vi "Initialize.vi"(8 "error in (no error)":errorcluster, 9 "Reset (T: Reset)":bool=TRUE, 10 "ID Query (T: Check)":bool=TRUE, 11 "VISA resource name":refnum<visa-resource-name>) -> (0 "error out":errorcluster, 3 "VISA resource name out":refnum<visa-resource-name>)   [LabVIEW 2015, in "Chroma ATE 6310.lvlib"]
doc: "This VI passes the addressing information in the instrument decriptor to the Instr Open VI and returns the instrument ID. You can optionally reset the instrument by setting the front panel reset control. You must run this VI before using any of the instrument driver VIs for this instrument."
uses:
  <instrlib>/Chroma ATE 6310/Chroma ATE 6310.lvlib
panel:
  # "© 2005 National Instruments.  ALL RIGHTS RESERVED."
  # "Check\nDon't Check"
  # "Reset\nDon't Reset"
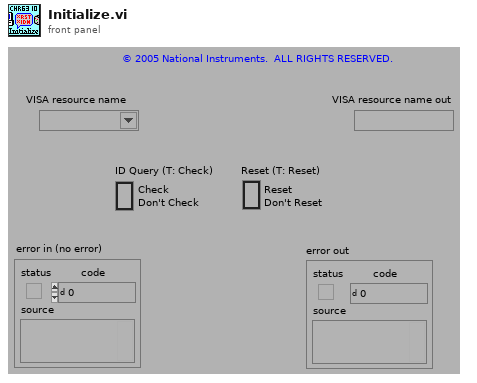
[diagram p1: front panel]
types:
  T1 = cluster{"Status":bool, "Code":i32, "Source (VI Name)":string}
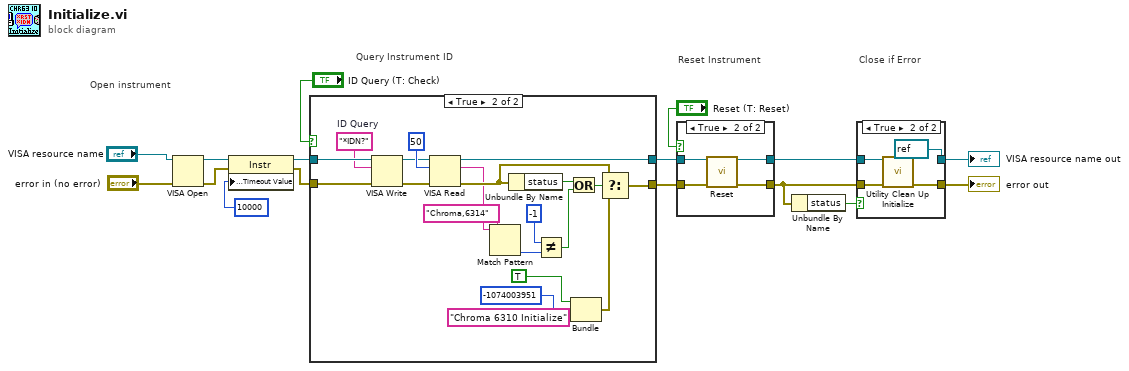
[diagram p0: block diagram]
diagram:
  # "Close if Error"
  # "Query Instrument ID"
  # "Reset Instrument"
  # "Open instrument"
  n1 = VISA Open(error in (no error)="error in (no error)", VISA resource name="VISA resource name") -> (VISA resource name=w3:refnum<visa-resource-name>, error out=w5:errorcluster)  [unwired: 3 in]
  n2 = property class="Instr"(reference=w3, error in=w5, "General Settings:Timeout Value"=u32 10000 ("Tmo Value")) -> (reference out=w2:refnum<visa-resource-name>, error out=w4:errorcluster)
  n3 = case shown="True" "ID Query (T: Check)" {
    tunnel: [w17 w38] -> w15
    tunnel: [w18 w35] -> w16
    tunnel: w2 -> [w18 w36]
    tunnel: w4 -> [w17 w37]
    frame False {
    }
    frame True {
      w31 = "*IDN?"  # ID Query
      n4 = VISA Write(VISA resource name=w36, write buffer=w31, error in (no error)=w37) -> (VISA resource name out=w22:refnum<visa-resource-name>, error out=w24:errorcluster)  [unwired: 1 out]
      n5 = VISA Read(VISA resource name=w22, byte count=u32 50, error in (no error)=w24) -> (VISA resource name out=w35:refnum<visa-resource-name>, read buffer=w21:string, error out=w23:errorcluster)  [unwired: 1 out]
      n6 = Match Pattern(string=w21, regular expression="Chroma,6314") -> (offset past match=w29:i32)  [unwired: 1 in, 3 out]
      n7 = Unbundle By Name(w23) -> ("status"=w26:bool)
      n8 = Not Equal?(x=-1, y=w29) -> (x != y?=w20:bool)
      n9 = Or(x=w26, y=w20) -> (x .or. y?=w25:bool)
      n10 = Bundle("Status"=TRUE, "Code"=-1074003951, "Source (VI Name)"="Chroma 6310 Initialize") -> (w32:T1)  [unwired: 1 in]
      n11 = Select(t=w23, s=w25, f=w32) -> (s? t:f=w38:T1)
    }
  }
  n12 = case shown="True" "Reset (T: Reset)" {
    tunnel: w15 -> [w39 w41]
    tunnel: [w39 w44] -> w10
    tunnel: w16 -> [w40 w42]
    tunnel: [w40 w43] -> w9
    frame False {
    }
    frame True {
      n13 = call <instrlib>:"Reset.vi"("VISA resource name"=w42, "error in (no error)"=w41) -> ("VISA resource name out"=w43:refnum<visa-resource-name>, "error out"=w44:errorcluster)  [unwired: 12 in]
    }
  }
  n14 = Unbundle By Name(w10) -> ("status"=w11:bool)
  n15 = case shown="True" w11 {
    tunnel: w9 -> [w46 w50]
    tunnel: w10 -> [w45 w49]
    tunnel: [w46 refnum<visa-resource-name> refnum ("VISA resource name out")] -> w8
    tunnel: [w45 w48] -> w7
    frame False {
    }
    frame True {
      n16 = call <instrlib>:"Utility Clean Up Initialize.vi"("VISA session"=w50, "error in (no error)"=w49) -> ("error out"=w48:errorcluster)  [unwired: 13 in]
    }
  }
  "VISA resource name out" <- w8
  "error out" <- w7
